vi "I-V扫描脚本.vi"(0 "扫描电压(V)":dbl, 1 "nplc":dbl, 2 "电压改变量":dbl, 3 "极限电流(mA)":dbl, 4 "时序优先":bool, 5 "时间点(ms)":dbl, 8 "4-wire":bool) -> (7 "Script":string)   [LabVIEW 2019]
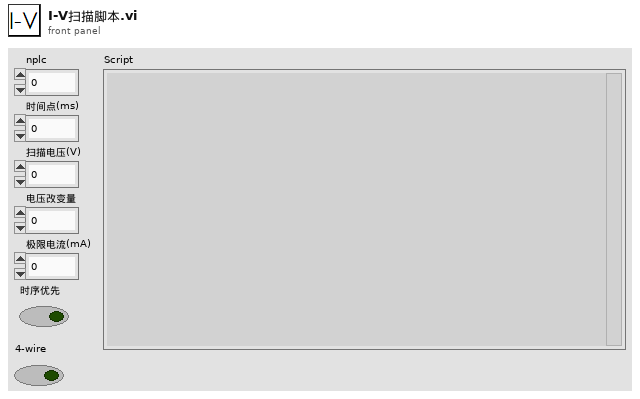
[diagram p1: front panel]
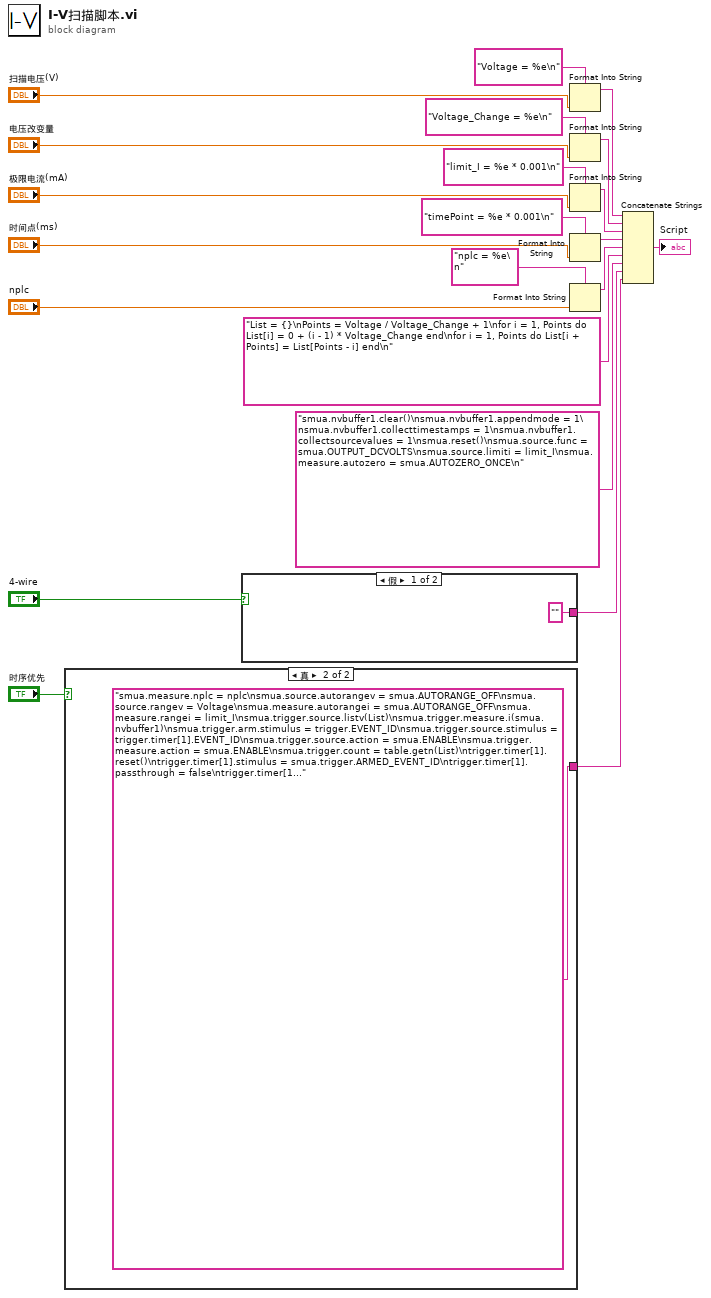
[diagram p0: block diagram]
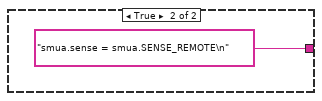
[diagram p2: hidden frame]
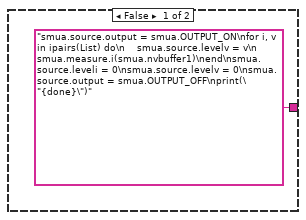
[diagram p3: hidden frame]
diagram:
  n1 = case shown="真" "时序优先" {
    tunnel: ["smua.source.output = smua.OUTPUT_ON\nfor i, v in ipairs(List) do\n    smua.source.levelv = v\n    smua.measure.i(smua.nvbuffer1)\nend\nsmua.source.leveli = 0\nsmua.source.levelv = 0\nsmua.source.output = smua.OUTPUT_OFF\nprint(\"{done}\")" "smua.measure.nplc = nplc\nsmua.source.autorangev = smua.AUTORANGE_OFF\nsmua.source.rangev = Voltage\nsmua.measure.autorangei = smua.AUTORANGE_OFF\nsmua.measure.rangei = limit_I\nsmua.trigger.source.listv(List)\nsmua.trigger.measure.i(smua.nvbuffer1)\nsmua.trigger.arm.stimulus = trigger.EVENT_ID\nsmua.trigger.source.stimulus = trigger.timer[1].EVENT_ID\nsmua.trigger.source.action = smua.ENABLE\nsmua.trigger.measure.action = smua.ENABLE\nsmua.trigger.count = table.getn(List)\ntrigger.timer[1].reset()\ntrigger.timer[1].stimulus = smua.trigger.ARMED_EVENT_ID\ntrigger.timer[1].passthrough = false\ntrigger.timer[1].delay = timePoint\ntrigger.timer[1].count = table.getn(List)\nsmua.source.output = smua.OUTPUT_ON\nsmua.trigger.initiate()\ndelay(1e-3)\nsmua.trigger.arm.set()\nfunction _done()\n    repeat\n        if (bit.test(status.operation.instrument.smua.condition, 4) == false) then\n            smua.source.leveli = 0\n            smua.source.levelv = 0\n            smua.source.output = smua.OUTPUT_OFF\n            print(\"{done}\")\n            return\n        end\n        delay(0.1)\n    until (false)\nend\n_done()"] -> w1
    frame False {
    }
    frame True {
    }
  }
  n2 = case shown="假" "4-wire" {
    tunnel: ["" "smua.sense = smua.SENSE_REMOTE\n"] -> w2
    frame False {
    }
    frame True {
    }
  }
  n3 = Format Into String(format string="Voltage = %e\n" ("格式字符串"), "扫描电压(V)") -> (resulting string=w17:string)  [unwired: 2 in, 1 out]
  n4 = Format Into String(format string="Voltage_Change = %e\n" ("格式字符串"), "电压改变量") -> (resulting string=w14:string)  [unwired: 2 in, 1 out]
  n5 = Format Into String(format string="limit_I = %e * 0.001\n" ("格式字符串"), "极限电流(mA)") -> (resulting string=w13:string)  [unwired: 2 in, 1 out]
  n6 = Format Into String(format string="timePoint = %e * 0.001\n", "时间点(ms)") -> (resulting string=w11:string)  [unwired: 2 in, 1 out]
  n7 = Format Into String(format string="nplc = %e\n", "nplc") -> (resulting string=w7:string)  [unwired: 2 in, 1 out]
  n8 = Concatenate Strings(w17, w14, w13, w11, w7, "List = {}\nPoints = Voltage / Voltage_Change + 1\nfor i = 1, Points do List[i] = 0 + (i - 1) * Voltage_Change end\nfor i = 1, Points do List[i + Points] = List[Points - i] end\n", "smua.nvbuffer1.clear()\nsmua.nvbuffer1.appendmode = 1\nsmua.nvbuffer1.collecttimestamps = 1\nsmua.nvbuffer1.collectsourcevalues = 1\nsmua.reset()\nsmua.source.func = smua.OUTPUT_DCVOLTS\nsmua.source.limiti = limit_I\nsmua.measure.autozero = smua.AUTOZERO_ONCE\n", w2, w1) -> (→"Script":string)
